vi "Represent Boolean.vi"(11 "String":string) -> (2 "Value":bool, 3 "Represent Boolean?":bool)   [LabVIEW 2020, in "hse-misc.lvlib"]
doc: "____\nHAMPEL SOFTWARE ENGINEERING v3.8.0 (2023-12-18 14:41)"
uses:
  hse-misc.lvlib
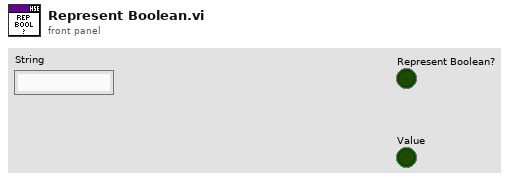
[diagram p1: front panel]
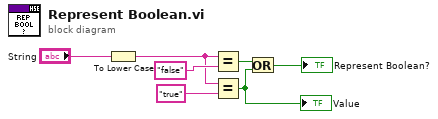
[diagram p0: block diagram]
diagram:
  n1 = To Lower Case(string="String") -> (all lower case string=w5:string)
  n2 = Equal?(x=w5, y="false" ("all lower case string")) -> (x = y?=w3:bool)
  n3 = Equal?(x=w5, y="true" ("all lower case string")) -> (x = y?=w2:bool)
  "Value" <- w2
  n4 = Or(x=w3, y=w2) -> (x .or. y?=→"Represent Boolean?":bool)
